vi "ts_tree_set_desc.vi"(8 "error in (no error)":errorcluster, 10 "ts.data":T1, 11 "Tree.in":refnum<vi>) -> (0 "error out":errorcluster, 3 "Tree.out":refnum<vi>)   [LabVIEW 2015]
doc: "sets the test step description in the tree control, ignares comments (#) and child test steps($)"
uses:
  ts-data.ctl
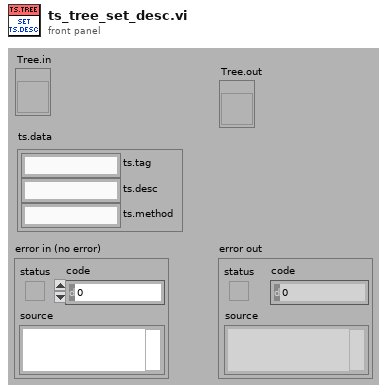
[diagram p1: front panel]
types:
  T1 = typedef "ts-data.ctl" = cluster{"ts.tag":string, "ts.desc":string, "ts.method":string}
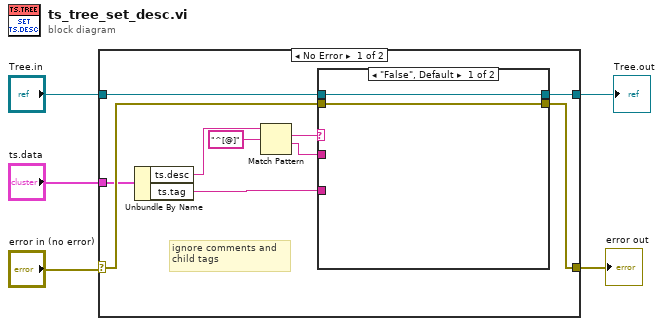
[diagram p0: block diagram]
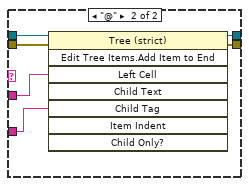
[diagram p2: hidden frame]
diagram:
  n1 = case shown="No Error" "error in (no error)" {
    selector: "error in (no error)" -> [w12 w24]
    tunnel: "Tree.in" -> [w15 w25]
    tunnel: [w14 w25] -> w3
    tunnel: [w11 w24] -> w2
    tunnel: "ts.data" -> [w10 _]
    frame No Error {
      # "ignore comments and\nchild tags"
      n2 = Unbundle By Name(w10) -> ("ts.desc"=w9:string, "ts.tag"=w13:string)
      n3 = Match Pattern(string=w9, regular expression="^[@]") -> (match substring=w7:string, after substring=w6:string)  [unwired: 1 in, 2 out]
      n4 = case shown="\"False\", Default" w7 {
        tunnel: w15 -> [w17 w23]
        tunnel: [w17 w22] -> w14
        tunnel: w6 -> [_ w21]
        tunnel: w13 -> [_ w20]
        tunnel: w12 -> [w16 w19]
        tunnel: [w16 w18] -> w11
        frame "False", Default {
        }
        frame "@" {
          n5 = invoke class="Tree (strict)" method="Edit Tree Items.Add Item to End"(reference=w23, error in=w19, "Left Cell"=w21, "Child Tag"=w20) -> (reference out=w22:refnum<vi>, error out=w18:errorcluster)  [unwired: 4 in, 6 out]
        }
      }
    }
    frame Error {
    }
  }
  "Tree.out" <- w3
  "error out" <- w2
